vi "VI Tree.vi"   [LabVIEW 2015, in "SDG X Series.lvlib"]
doc: "This is the instrument driver for the Siglent SDG X series function(Pulse)/arbitrary generators. The VI Tree displays all the user-callable VIs of the instrument driver in an organized table."
uses:
  <instrlib>/SDG X Series/SDG X Series.lvlib
  <instrlib>/SDG X Series/Public/Configure/Configure Modulation (AM).vi
panel:
  # "(c) 2017 SIGLENT TECHNOLOGIES CO.,LTD. ALL RIGHTS RESERVED."
  # "SEE DIAGRAM\nFOR VI TREE."
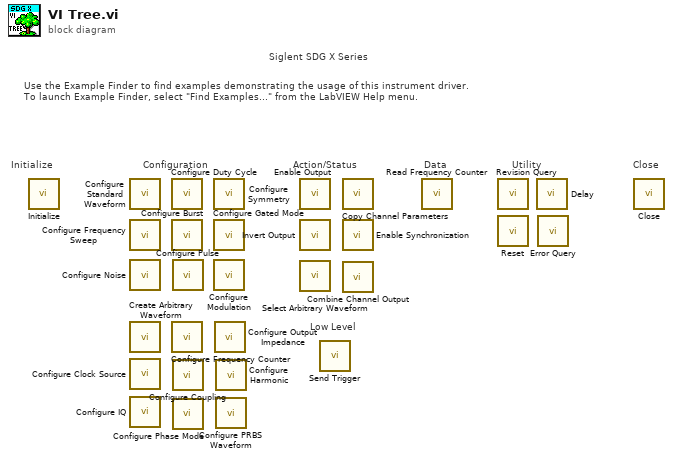
[diagram p0: block diagram]
diagram:
  # "Siglent SDG X Series"
  # "Data"
  # "Low Level"
  # "Use the Example Finder to find examples demonstrating the usage of this instrument driver.\nTo launch Example Finder, select \"Find Examples...\" from the LabVIEW Help menu."
  # "Configuration"
  # "Utility"
  # "Action/Status"
  # "Close"
  # "Initialize"
  n1 = call <instrlib>:"Initialize.vi"() -> ()  [unwired: 10 in, 2 out]
  n2 = call <instrlib>:"Configure Standard Waveform.vi"() -> ()  [unwired: 14 in, 2 out]
  n3 = call <instrlib>:"Configure Frequency Sweep.vi"() -> ()  [unwired: 14 in, 2 out]
  n4 = call <instrlib>:"Configure Noise.vi"() -> ()  [unwired: 10 in, 2 out]
  n5 = call <instrlib>:"Create Arbitrary Waveform.vi"() -> ()  [unwired: 10 in, 2 out]
  n6 = call <instrlib>:"Configure Clock Source.vi"() -> ()  [unwired: 10 in, 2 out]
  n7 = call <instrlib>:"Configure IQ.vi"() -> ()  [unwired: 14 in, 2 out]
  n8 = call <instrlib>:"Configure Duty Cycle.vi"() -> ()  [unwired: 10 in, 2 out]
  n9 = call <instrlib>:"Configure Burst.vi"() -> ()  [unwired: 18 in, 2 out]
  n10 = call <instrlib>:"Configure Frequency Counter.vi"() -> ()  [unwired: 10 in, 2 out]
  n11 = call <instrlib>:"Configure Pulse.vi"() -> ()  [unwired: 10 in, 2 out]
  n12 = call <instrlib>:"Configure Coupling.vi"() -> ()  [unwired: 10 in, 2 out]
  n13 = call <instrlib>:"Configure Phase Mode.vi"() -> ()  [unwired: 10 in, 2 out]
  n14 = call <instrlib>:"Configure Symmetry.vi"() -> ()  [unwired: 10 in, 2 out]
  n15 = call <instrlib>:"Configure Gated Mode.vi"() -> ()  [unwired: 10 in, 2 out]
  n16 = call-poly <instrlib>:"Configure Modulation.vi"() -> ()  [unwired: 10 in, 2 out]
  n17 = call <instrlib>:"Configure Output Impedance.vi"() -> ()  [unwired: 10 in, 2 out]
  n18 = call <instrlib>:"Configure Harmonic.vi"() -> ()  [unwired: 14 in, 2 out]
  n19 = call <instrlib>:"Configure PRBS Waveform.vi"() -> ()  [unwired: 10 in, 2 out]
  n20 = call <instrlib>:"Enable Output.vi"() -> ()  [unwired: 10 in, 2 out]
  n21 = call <instrlib>:"Invert Output.vi"() -> ()  [unwired: 10 in, 2 out]
  n22 = call <instrlib>:"Select Arbitrary Waveform.vi"() -> ()  [unwired: 10 in, 2 out]
  n23 = call <instrlib>:"Send Trigger.vi"() -> ()  [unwired: 10 in, 2 out]
  n24 = call <instrlib>:"Copy Channel Parameters.vi"() -> ()  [unwired: 10 in, 2 out]
  n25 = call <instrlib>:"Enable Synchronization.vi"() -> ()  [unwired: 10 in, 2 out]
  n26 = call <instrlib>:"Combine Channel Output.vi"() -> ()  [unwired: 10 in, 2 out]
  n27 = call <instrlib>:"Read Frequency Counter.vi"() -> ()  [unwired: 5 in, 7 out]
  n28 = call <instrlib>:"Revision Query.vi"() -> ()  [unwired: 8 in, 4 out]
  n29 = call <instrlib>:"Reset.vi"() -> ()  [unwired: 10 in, 2 out]
  n30 = call <instrlib>:"Delay.vi"() -> ()  [unwired: 10 in, 2 out]
  n31 = call <instrlib>:"Error Query.vi"() -> ()  [unwired: 8 in, 4 out]
  n32 = call <instrlib>:"Close.vi"() -> ()  [unwired: 11 in, 1 out]
